vi "XYAdd-.vi"(7 "枚举":enum16{"insert", "add", "read", "reset"}(ring), 9 "数据":cluster{dbl[], dbl[]}[](array[cluster]), 10 "position":u32, 11 "XYGraph":refnum<vi>) -> (1 "XYData":cluster{dbl[], dbl[]}[](array[cluster]), 3 "XYGraph 2":refnum<vi>)   [LabVIEW 2019]
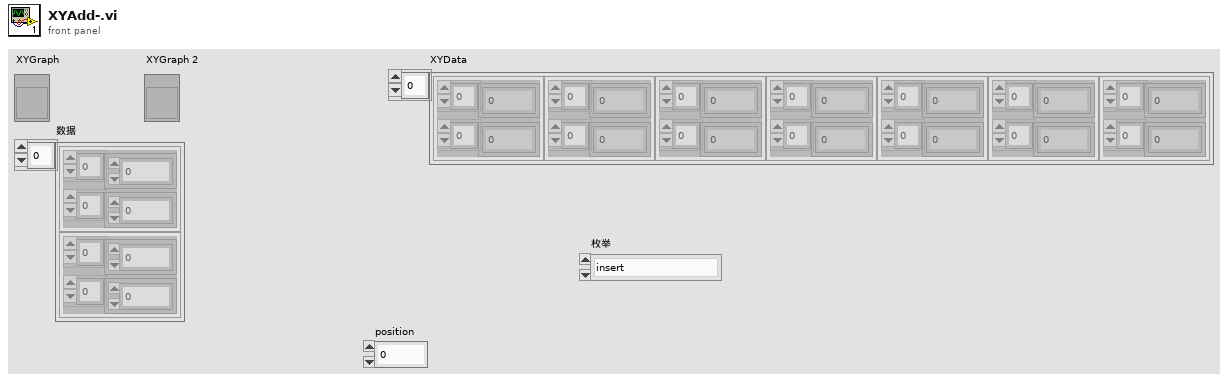
[diagram p1: front panel]
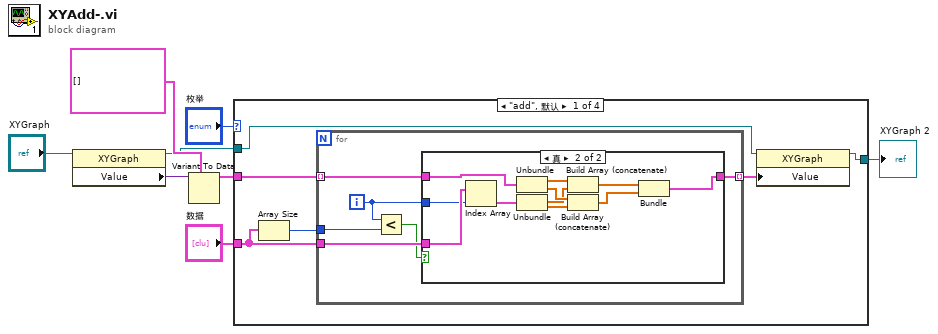
[diagram p0: block diagram]
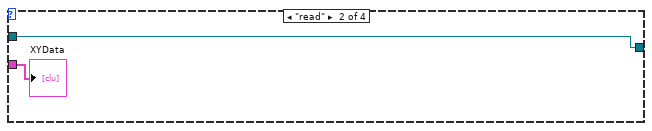
[diagram p3: hidden frame]
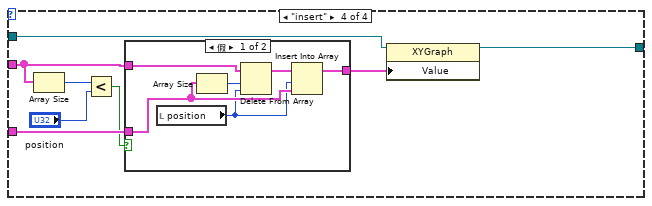
[diagram p5: hidden frame]
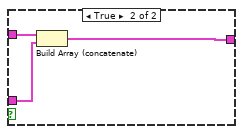
[diagram p6: hidden frame]
diagram:
  n1 = property class="XYGraph"(reference="XYGraph") -> (reference out=w1:refnum<vi>, "Value"=w6:variant)  [unwired: 1 in, 1 out]
  n2 = Variant To Data(type=cluster{dbl[], dbl[]}[] [] ("添加的数组"), Variant=w6) -> (data=w5:cluster{dbl[], dbl[]}[])  [unwired: 1 in, 1 out]
  n3 = case shown="\"add\", 默认" "枚举" {
    tunnel: w1 -> [w12 w34 w35 w42]
    tunnel: [w13 w34 w35 w41] -> w7
    tunnel: w5 -> [w11 w33 _ w39]
    tunnel: "数据" -> [w10 _ _ w40]
    frame "add", Default {
      n4 = Array Size(array=w10) -> (size(s)=w9:i32)
      n5 = for {
        tunnel: w11 -> [w19] mode=indexing
        tunnel: [w20] -> w14 mode=indexing
        tunnel: w10 -> [w18]
        tunnel: w9 -> [w16]
        i -> [w17]
        n6 = Less?(x=w17, y=w16) -> (x < y?=w15:bool)
        n7 = case shown="真" w15 {
          tunnel: [w21 w32] -> w20
          tunnel: w19 -> [w21 w31]
          tunnel: w18 -> [_ w23]
          tunnel: w17 -> [_ w22]
          frame False {
          }
          frame True {
            n8 = Index Array(array=w23, index=w22) -> (element=w24:cluster{dbl[], dbl[]})
            n9 = Unbundle(w31) -> (w30:dbl[], w29:dbl[])
            n10 = Unbundle(w24) -> (w26:dbl[], w25:dbl[])
            n11 = Build Array (concatenate)(w30, w26) -> (w28:dbl[])
            n12 = Build Array (concatenate)(w29, w25) -> (w27:dbl[])
            n13 = Bundle(w28, w27) -> (w32:cluster{dbl[], dbl[]})  [unwired: 1 in]
          }
        }
      }
      n14 = property class="XYGraph"(reference=w12, "Value"=w14) -> (reference out=w13:refnum<vi>)  [unwired: 1 in, 1 out]
    }
    frame "read" {
      "XYData" <- w33
    }
    frame "reset" {
    }
    frame "insert" {
      n15 = Array Size(array=w39) -> (size(s)=w38:i32)
      n16 = Less?(x=w38, y="position") -> (x < y?=w36:bool)
      n17 = case shown="假" w36 {
        tunnel: [w49 w50] -> w43
        tunnel: w39 -> [w48 w52]
        tunnel: w40 -> [w47 w51]
        frame False {
          n18 = local read "position"() -> (w45:u32)
          n19 = Array Size(array=w47) -> (size(s)=w46:i32)
          n20 = Delete From Array(array=w48, length=w46, index=w45) -> (array with subset deleted=w44:cluster{dbl[], dbl[]}[])  [unwired: 1 out]
          n21 = Insert Into Array(array=w44, index=w45, new element=w47) -> (w49:cluster{dbl[], dbl[]}[])
        }
        frame True {
          n22 = Build Array (concatenate)(w52, w51) -> (w50:cluster{dbl[], dbl[]}[])
        }
      }
      n23 = property class="XYGraph"(reference=w42, "Value"=w43) -> (reference out=w41:refnum<vi>)  [unwired: 1 in, 1 out]
    }
  }
  "XYGraph 2" <- w7
